vi "Convert Step to Report Line.vi"(9 "Report Data":T1, 11 "Step":T2) -> (3 "Report Line":string)   [LabVIEW 2020, in "MacroAssert.lvlib"]
uses:
  MacroAssert.lvlib
  CTLs/Step Type V3.ctl
  CTLs/Assertion Type.ctl
  CTLs/Step V3.ctl
  CTLs/Report Data.ctl
  <vilib>/picture/picture.llb/imagedata.ctl
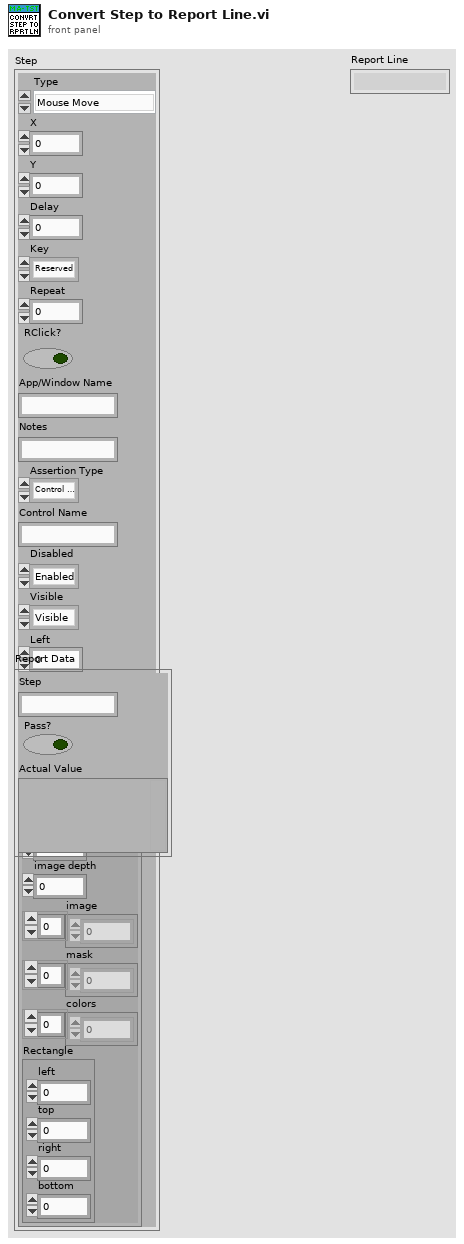
[diagram p1: front panel]
types:
  T1 = typedef "MacroAssert.lvlib/Report Data.ctl" = cluster{"Step":string, "Pass?":bool, "Actual Value":variant}
  T2 = typedef "MacroAssert.lvlib/Step V3.ctl" = cluster{"Type":T3, "X":i32, "Y":i32, "Delay":i32, "Key":u8, "Repeat":i32, "RClick?":bool, "App/Window Name":string, "Notes":string, "Assertion Type":T4, "Control Name":string, "Disabled":enum8{"Enabled", "Disabled", "Disabled and Grayed Out"}, "Visible":enum16{"Visible", "Not Visible"}, "Left":i16, "Top":i16, "Width":i16, "Height":i16, "Expected Image":T5}
  T3 = typedef "MacroAssert.lvlib/Step Type V3.ctl" = enum16{"Mouse Move", "Mouse Click", "Key Press", "Wait", "Mouse Down", "Mouse Up", "Key Down", "Key Up", "Test Assertion", "Run Application", "Maximize Window", "Restore Window", "Minimize Window", "Close Window", "Bring Window to Front", "Send Window to Back"}
  T4 = typedef "MacroAssert.lvlib/Assertion Type.ctl" = enum16{"Control Position", "Control Visible", "Control Disabled", "Control Image"}
  T5 = typedef "imagedata.ctl" = cluster{"image type":i32, "image depth":i32, "image":u8[], "mask":u8[], "colors":u32[], "Rectangle":cluster{"left":i16, "top":i16, "right":i16, "bottom":i16}}
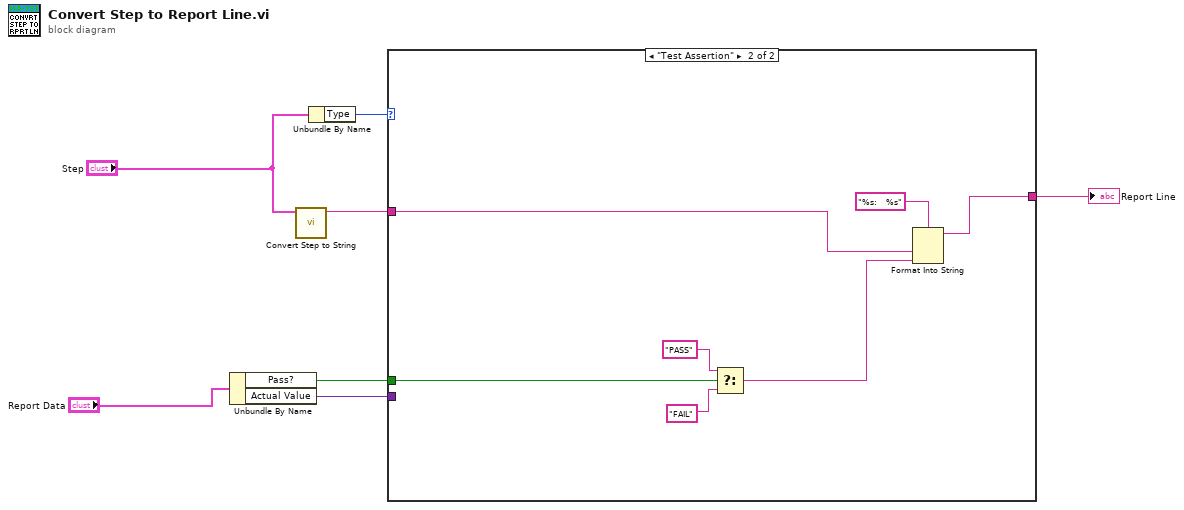
[diagram p0: block diagram]
diagram:
  n1 = Unbundle By Name("Report Data") -> ("Pass?"=w5:bool, "Actual Value"=w4:variant)
  n2 = call "Convert Step to String.vi"("Step"="Step") -> ("Step String"=w1:string)  [unwired: 10 in]
  n3 = Unbundle By Name("Step") -> ("Type"=w7:T3)
  n4 = case shown="\"Test Assertion\"" w7 {
    tunnel: w5 -> [_ w15]
    tunnel: w4 -> [_ _]
    tunnel: [w8 w10] -> w3
    tunnel: w1 -> [w8 w9]
    frame "Mouse Move", Default {
    }
    frame "Test Assertion" {
      n5 = Select(t="PASS", s=w15, f="FAIL") -> (s? t:f=w11:string)
      n6 = Format Into String(format string="%s:   %s", w9, w11) -> (resulting string=w10:string)  [unwired: 2 in, 1 out]
    }
  }
  "Report Line" <- w3
